vi "Clear-object.vi"(8 "error in (no error)":errorcluster, 11 "Reference in":T1) -> (0 "error out":errorcluster)   [LabVIEW 2013, in "HardwareCharacterization.lvlib" / "HC-ScanParser.lvclass"]
uses:
  HC-ScanParser.lvclass
  Object-reference.ctl
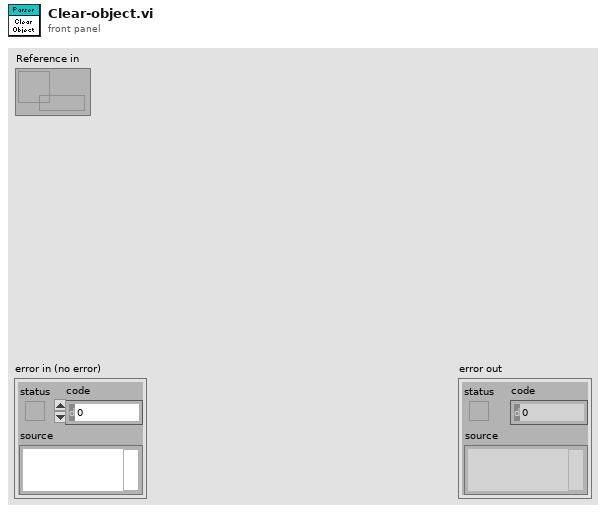
[diagram p1: front panel]
types:
  T1 = typedef "HardwareCharacterization.lvlib/HC-ScanParser.lvclass/Object-reference.ctl" = refnum<data-value>
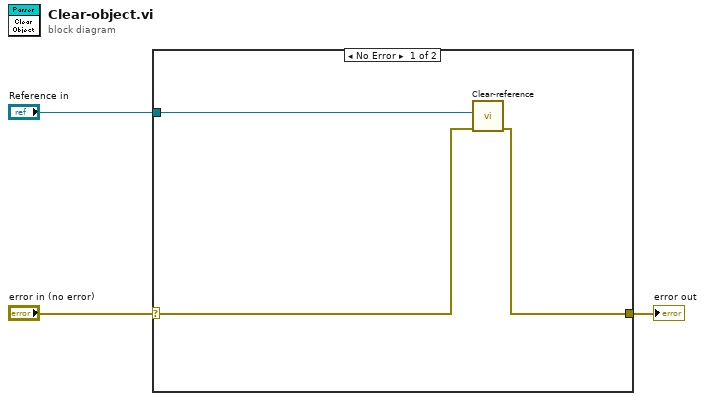
[diagram p0: block diagram]
diagram:
  n1 = case shown="No Error" "error in (no error)" {
    selector: "error in (no error)" -> [w4 w7]
    tunnel: [w6 w7] -> w2
    tunnel: "Reference in" -> [w5 _]
    frame No Error {
      n2 = call "Clear-reference.vi"("error in (no error)"=w4, "Object reference"=w5) -> ("error out"=w6:errorcluster)  [unwired: 8 in, 1 out]
    }
    frame Error {
    }
  }
  "error out" <- w2
